vi "Get GUI Item Ref.vi"(8 "error in (no error)":errorcluster, 10 "FP Item Name":string, 11 "uService Template in":refnum<class "Father of all uServices.lvclass">) -> (0 "error out":errorcluster, 2 "Ctl Refnum":refnum<vi>, 3 "uService Template out":refnum<class "Father of all uServices.lvclass">)   [LabVIEW 2026, in "TALOS.lvlib" / "Father of all uServices.lvlib" / "Father of all uServices.lvclass"]
doc: "This VI gives the Ref of the uService GUI Item given in input."
uses:
  Father of all uServices.lvclass
  C:/LabVIEW Code/TALOS/talos/Ancestor/Ancestor/Ancestor.lvclass
  Ancestor/Ancestor/Ancestor.lvclass/Ancestor.ctl
  Classes/uService List/uService List.lvclass/uService List.ctl
  Classes/uService List/Get FP Items Refs Map.vi
  Ancestor/Ancestor/Read ID.vi
  FGV/Error Memory/Get Error Description.vi
  Support VIs/Get PC name.vi
  Support VIs/Get Class Name.vi
  <vilib>/Utility/error.llb/Clear Errors.vi
  FGV/Error Memory/Error Memory Core.vi
  <vilib>/AdvancedString/Delimited String to 1D String Array.vi
  <vilib>/AdvancedString/Delimited String to 1D String Array (string).vi
  Support VIs/Circus Root Path.vi
  FGV/Error Memory/Error Crt Lvl checker.vi
  FGV/Error Memory/Error Memory Core.vi/40c8088d-b597-4017-91af-faa98e00292e.vi
  FGV/Error Memory/Error Memory Core.vi/d4a3ab98-063c-4e44-b43d-fbdcfe6c2be2.vi
  Support VIs/Global Memory.vi
  <vilib>/Utility/LVClass/Get LV Class Name.vi
  Support VIs/Is in Packed Library.vi
  Support VIs/TALOS Root path.vi
  Support VIs/Read CSV worksheet.vi
  Support VIs/Global Constants.vi
  <vilib>/Utility/error.llb/General Error Handler.vi
  Ancestor/Ancestor/Ancestor.lvclass
  <vilib>/Comparison/Equal/Equal Functor/Equal Functor.lvclass
  Classes/uService List/uService List.lvclass
  TALOS.lvlib
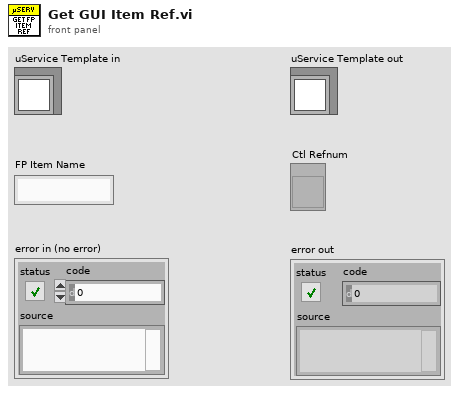
[diagram p1: front panel]
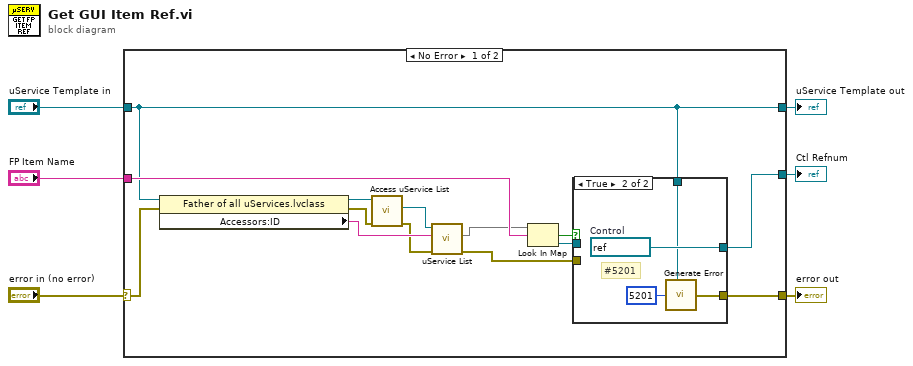
[diagram p0: block diagram]
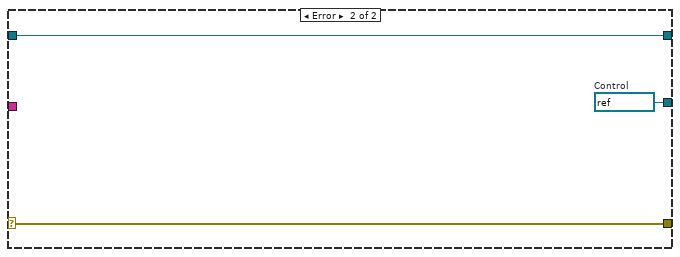
[diagram p3: hidden frame]
diagram:
  n1 = case shown="No Error" "error in (no error)" {
    selector: "error in (no error)" -> [w16 w29]
    tunnel: "uService Template in" -> [w11 w28]
    tunnel: [w18 w27] -> w1
    tunnel: "FP Item Name" -> [w17 _]
    tunnel: [w15 w29] -> w3
    tunnel: [w11 w28] -> w2
    frame No Error {
      n2 = property class="Father of all uServices.lvclass"(reference=w11, error in=w16) -> (reference out=w12:refnum<class "Father of all uServices.lvclass">, error out=w10:errorcluster, "Accessors:ID"=w13:string)
      n3 = call-dynamic "Access uService List.vi"("error in (no error)"=w10, "Ancestor in"=w12) -> ("error out"=w9:errorcluster, "uService List out"=w8:refnum<class "uService List.lvclass">)  [unwired: 7 in, 1 out]
      n4 = call-poly "uService List.vi"("error in (no error)"=w9, "ID"=w13, "uService List in"=w8) -> ("error out"=w14:errorcluster, "FP Items Refs Map"=w7:map{string, refnum<vi>})  [unwired: 6 in, 1 out]
      n5 = Look In Map(map=w7, key=w17) -> (key not found?=w19:bool, value=w20:refnum<vi>)  [unwired: 1 in]
      n6 = case shown="True" w19 {
        tunnel: w20 -> [w22 _]
        tunnel: w14 -> [w21 _]
        tunnel: [w21 w25] -> w15
        tunnel: [w22 w26] -> w18
        tunnel: w11 -> [_ w24]
        frame False {
          # "Key found"
        }
        frame True {
          w26 = refnum<vi> refnum  # Control
          # "#5201"
          n7 = call "Generate Error.vi"("Class"=w24, "Error Code"=5201) -> ("error out"=w25:errorcluster)  [unwired: 5 in]
        }
      }
    }
    frame Error {
      w27 = refnum<vi> refnum  # Control
    }
  }
  "error out" <- w3
  "uService Template out" <- w2
  "Ctl Refnum" <- w1
